vi "DO Create.vi"(8 "error in (no error)":errorcluster, 10 "Digital Configuration Parameters":T1, 11 "Binary Valve in":refnum<class "Binary Valve.lvclass">) -> (0 "error out":errorcluster, 3 "Binary Valve out":refnum<class "Binary Valve.lvclass">)   [LabVIEW 2021, in "Binary Valve.lvlib" / "Binary Valve.lvclass"]
uses:
  Binary Valve.lvclass
  Binary Valve.lvclass/Binary Valve.ctl
  <vilib>/NathanCo/Digital Tasks/Digital Output/Digital Output/Digital Output.lvclass
  <vilib>/NathanCo/Digital Tasks/Utilities/Digital Configuration Parameters.ctl
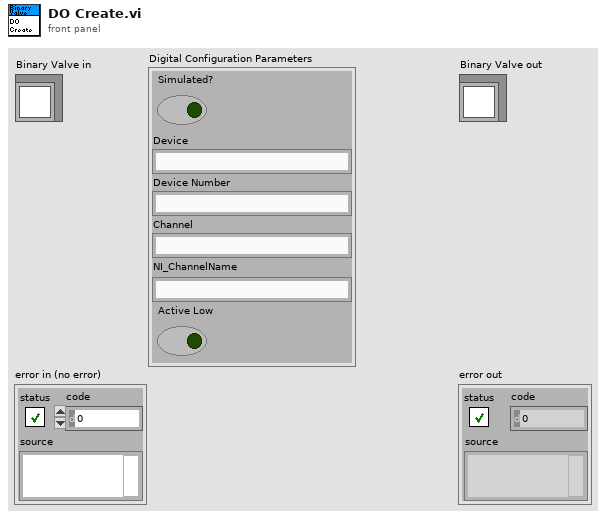
[diagram p1: front panel]
types:
  T1 = typedef "Digital Configuration Parameters.ctl" = cluster{"Simulated?":bool, "Device":string, "Device Number":string, "Channel":string, "NI_ChannelName":string, "Active Low":bool}
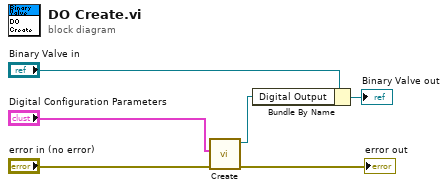
[diagram p0: block diagram]
diagram:
  n1 = call <vilib>:"Create.vi"("error in (no error)"="error in (no error)", "Digital Configuration Parameters"="Digital Configuration Parameters") -> ("error out"=→"error out":errorcluster, "Digital Output out"=w2:refnum<class "Digital Output.lvclass">)  [unwired: 8 in]
  n2 = Bundle By Name(cluster="Binary Valve in", "Digital Output"=w2) -> (→"Binary Valve out":refnum<class "Binary Valve.lvclass">)
